vi "Build Display Array.vi"(6 "Status":string, 9 "Notes":string, 10 "Name":string) -> (2 "Display Array":string[](array[string]), 3 "Spreadsheet String":string)   [LabVIEW 2020]
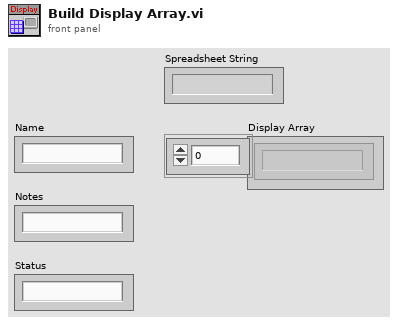
[diagram p1: front panel]
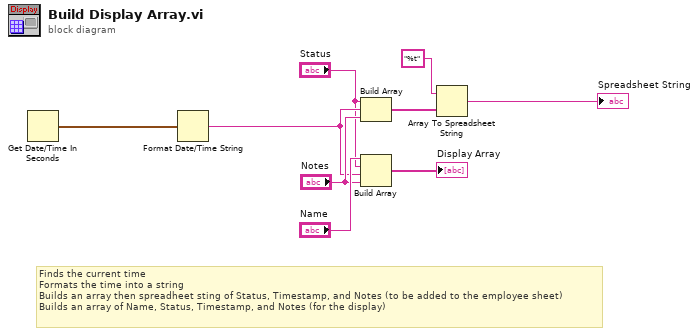
[diagram p0: block diagram]
diagram:
  # "Finds the current time\nFormats the time into a string\nBuilds an array then spreadheet sting of Status, Timestamp, and Notes (to be added to the employee sheet)\nBuilds an array of Name, Status, Timestamp, and Notes (for the display)"
  n1 = Get Date/Time In Seconds() -> (seconds since 1Jan1904=w2:timestamp)
  n2 = Format Date/Time String(seconds (now)=w2) -> (date/time string=w4:string)  [unwired: 2 in]
  n3 = Build Array "Build Array"("Status", w4, "Notes") -> (w7:string[])
  n4 = Build Array "Build Array"("Name", "Status", w4, "Notes") -> (→"Display Array":string[])
  n5 = Array To Spreadsheet String(array=w7, 3:"%t" ("format string")) -> (spreadsheet string=→"Spreadsheet String":string)  [unwired: 1 in]
